vi "MODEL SELECTION.vi"(8 "error in (no error)":errorcluster, 11 "Plan List":string[](array[string])) -> (0 "error out 2":errorcluster, 3 "Plan Selected":string(combo))   [LabVIEW 2017]
panel:
  in  "RECIPE SELECT":string(combo)
  in  "Cancel Button":bool
  in  "Save Button":bool
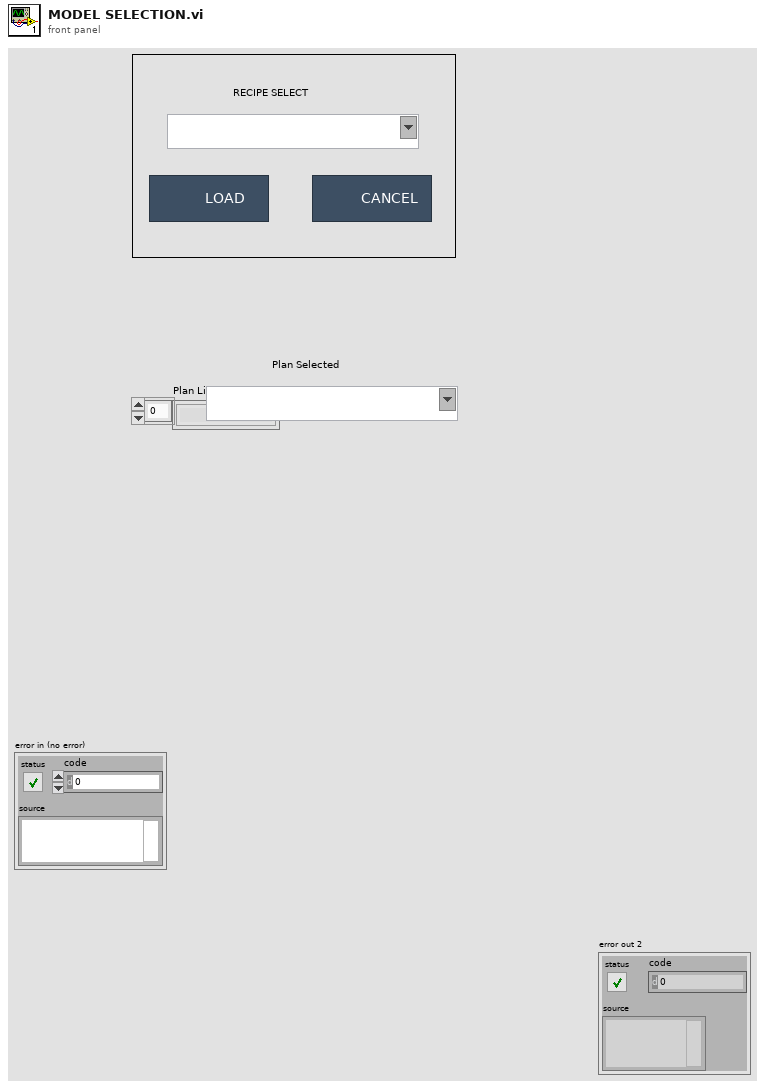
[diagram p1: front panel]
types:
  T1 = enum32{"invalid app kind", "Development System", "Run Time System", "Student Edition", "Embedded LabVIEW", "Evaluation", "Custom"}
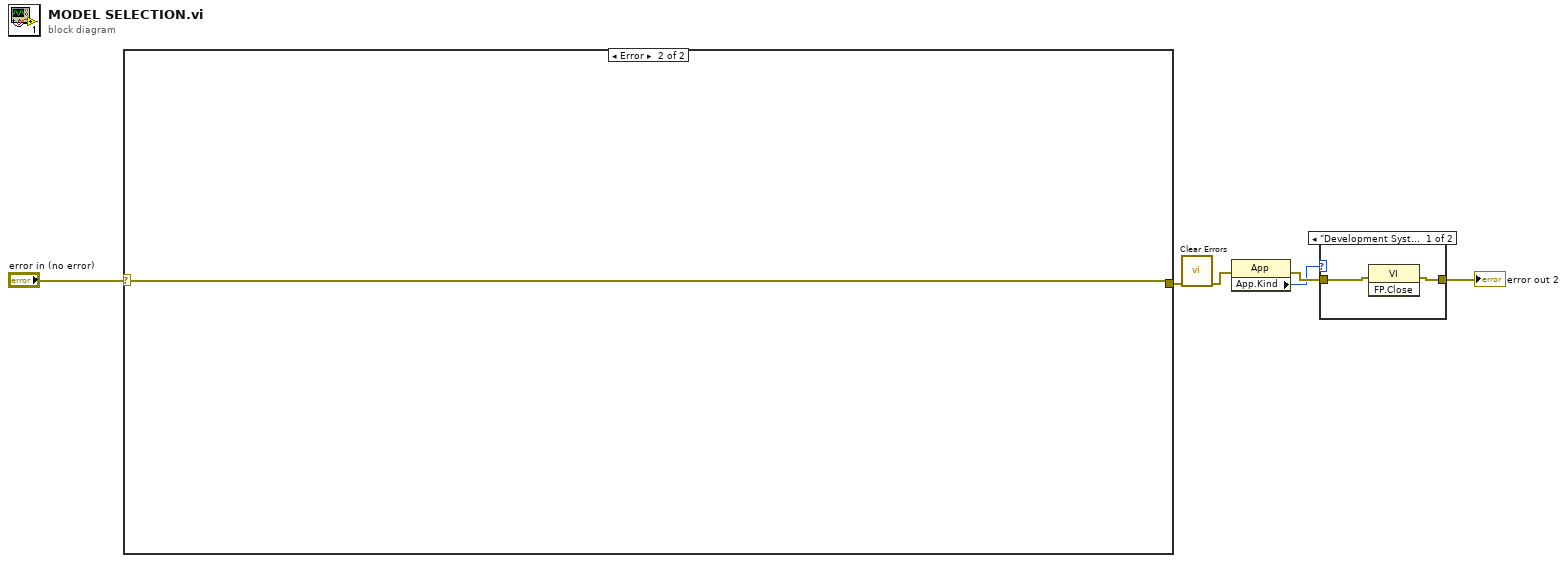
[diagram p0: block diagram]
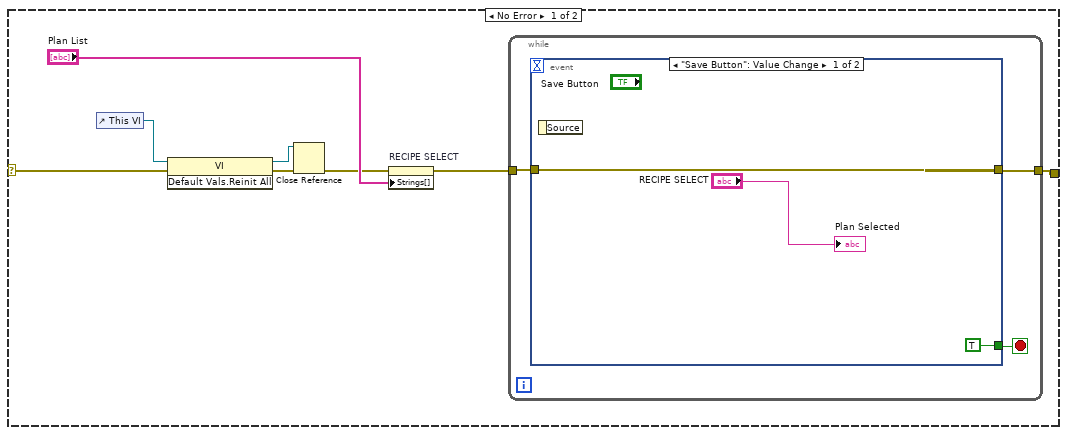
[diagram p2: hidden frame]
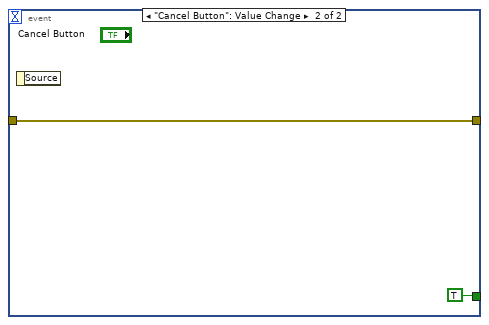
[diagram p3: hidden frame]
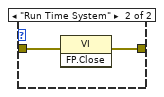
[diagram p4: hidden frame]
diagram:
  n1 = case shown="Error" "error in (no error)" {
    selector: "error in (no error)" -> [w12 w23]
    tunnel: [w14 w23] -> w6
    frame No Error {
      n2 = control-ref of="This VI"() -> (w13:refnum<vi>)
      n3 = invoke class="VI" method="Default Vals.Reinit All"(reference=w13, error in=w12) -> (reference out=w11:refnum<vi>, error out=w10:errorcluster)  [unwired: 1 in, 1 out]
      n4 = Close Reference(reference=w11, error in (no error)=w10) -> (error out=w7:errorcluster)
      n5 = property on="RECIPE SELECT" class="CmbBox"(error in=w7, "Strings[]"="Plan List") -> (error out=w8:errorcluster)  [unwired: 1 in, 1 out]
      n6 = while {
        tunnel: w8 -> [w15]
        tunnel: [w16] -> w14
        stop <- w17 stop-if-true
        n7 = event shown="[0] \"Save Button\": Value Change" {
          selector: _ -> [_ _]
          dyn-events: _ -> [_ _]
          timeout: _ -> [_ _]
          tunnel: [TRUE TRUE] -> w17
          tunnel: [w19 w21] -> w16
          tunnel: w15 -> [w19 w21]
          event "Save Button": Value Change {
            n8 = event-data() -> ()  [unwired: 1 in, 1 out]
            "Plan Selected" <- "RECIPE SELECT"
          }
          event "Cancel Button": Value Change {
            n9 = event-data() -> ()  [unwired: 1 in, 1 out]
          }
        }
      }
    }
    frame Error {
    }
  }
  n10 = call <vilib>:"Clear Errors.vi"("error in (no error)"=w6) -> ("error out"=w1:errorcluster)  [unwired: 5 in, 1 out]
  n11 = property class="App"(error in=w1) -> (error out=w3:errorcluster, "App.Kind"=w2:T1)  [unwired: 1 in, 1 out]
  n12 = case shown="\"Development System\", Default" w2 {
    tunnel: [w24 w27] -> w4
    tunnel: w3 -> [w25 w26]
    frame "Development System", Default {
      n13 = invoke class="VI" method="FP.Close"(error in=w25) -> (error out=w24:errorcluster)  [unwired: 2 in, 2 out]
    }
    frame "Run Time System" {
      n14 = invoke class="VI" method="FP.Close"(error in=w26) -> (error out=w27:errorcluster)  [unwired: 2 in, 2 out]
    }
  }
  "error out 2" <- w4
